vi "12_NODO_COVID_19.vi"() -> ()   [LabVIEW 2019]
panel:
  in  "Knob":u8(knob) scale=0.0..100.0
  in  "INTRODUZCA LA CLAVE":string
  in  "POSICIÓN":bool
  in  "PARPADEO":bool
  in  "COLOR":bool
  in  "stop":bool
  out "LED_ALARMA":bool
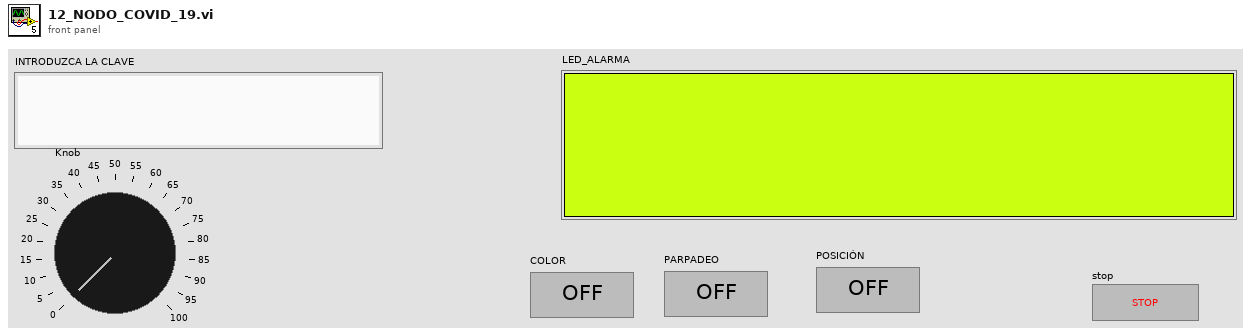
[diagram p1: front panel]
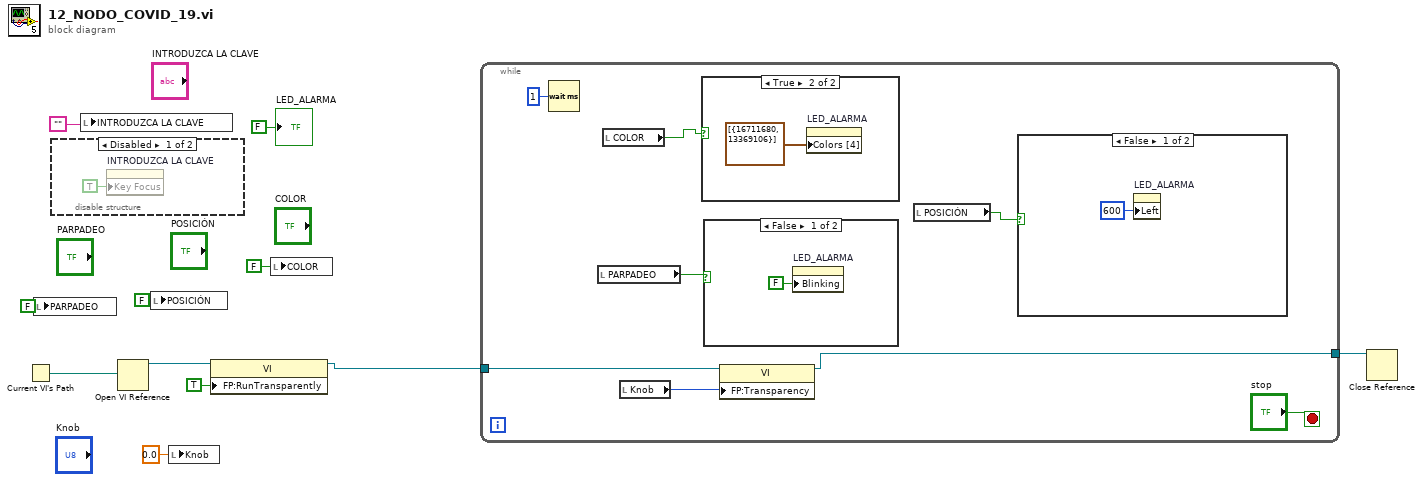
[diagram p0: block diagram]
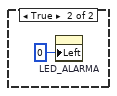
[diagram p3: hidden frame]
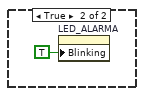
[diagram p4: hidden frame]
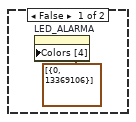
[diagram p5: hidden frame]
diagram:
  n1 = Current VI's Path() -> (path=w6:path)
  n2 = local write "PARPADEO"(FALSE ("COLOR")) -> ()
  n3 = disable-structure shown="Disabled" {
    frame Disabled {
      n4 = property on="INTRODUZCA LA CLAVE" class="Str"("Key Focus"=TRUE) -> ()  [unwired: 2 in, 2 out]
    }
    frame Enabled {
    }
  }
  n5 = local write "INTRODUZCA LA CLAVE"("") -> ()
  n6 = Open VI Reference(vi path=w6) -> (vi reference=w5:refnum<vi>)  [unwired: 5 in, 1 out]
  n7 = local write "POSICIÓN"(FALSE ("COLOR")) -> ()
  n8 = local write "Knob"(0.0 ("Knob")) -> ()
  n9 = property class="VI"(reference=w5, "FP:RunTransparently"=TRUE ("Front Panel Window:Run VI Transparently")) -> (reference out=w3:refnum<vi>)  [unwired: 1 in, 1 out]
  n10 = local write "COLOR"(FALSE ("COLOR")) -> ()
  n11 = while {
    tunnel: w3 -> [w15]
    tunnel: [w13] -> w2
    stop <- "stop" stop-if-true
    n12 = Wait (ms)(milliseconds to wait=u32 1) -> ()  [unwired: 1 out]
    n13 = local read "PARPADEO"() -> (w17:bool)
    n14 = local read "COLOR"() -> (w18:bool)
    n15 = local read "Knob"() -> (w14:u8)
    n16 = case shown="True" w18 {
      frame False {
        n17 = property on="LED_ALARMA" class="Bool (strict)"("Colors [4]"=cluster{u32, u32}[] [{0, 13369106}] ("Colors [4] 2")) -> ()  [unwired: 2 in, 2 out]
      }
      frame True {
        n18 = property on="LED_ALARMA" class="Bool (strict)"("Colors [4]"=cluster{u32, u32}[] [{16711680, 13369106}]) -> ()  [unwired: 2 in, 2 out]
      }
    }
    n19 = case shown="False" w17 {
      frame False {
        n20 = property on="LED_ALARMA" class="Bool (strict)"("Blinking"=FALSE) -> ()  [unwired: 2 in, 2 out]
      }
      frame True {
        n21 = property on="LED_ALARMA" class="Bool (strict)"("Blinking"=TRUE) -> ()  [unwired: 2 in, 2 out]
      }
    }
    n22 = property class="VI"(reference=w15, "FP:Transparency"=w14) -> (reference out=w13:refnum<vi>)  [unwired: 1 in, 1 out]
    n23 = local read "POSICIÓN"() -> (w16:bool)
    n24 = case shown="False" w16 {
      frame False {
        n25 = property on="LED_ALARMA" class="Bool (strict)"("Left"=600 ("Position:Left")) -> ()  [unwired: 2 in, 2 out]
      }
      frame True {
        n26 = property on="LED_ALARMA" class="Bool (strict)"("Left"=0 ("Position:Left")) -> ()  [unwired: 2 in, 2 out]
      }
    }
  }
  n27 = Close Reference(reference=w2) -> ()  [unwired: 1 in, 1 out]
  "LED_ALARMA" <- FALSE ("Boolean")
